vi "Update Conditional Visibility.vi"(10 "Previous UI Data in":refnum<class "Settings UI.lvclass">, 11 "New UI Data in":refnum<class "Settings UI.lvclass">) -> (3 "New UI Data out":refnum<class "Settings UI.lvclass">)   [LabVIEW 2024, in "Output Sequencer.lvlib" / "Settings UI.lvclass"]
uses:
  Settings UI.lvclass
  Types/Tree Index Enum.ctl
  Settings UI.lvclass/Settings UI.ctl
  Globals/Global Tree Data.vi
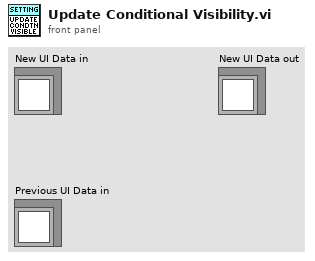
[diagram p1: front panel]
types:
  T1 = typedef "Output Sequencer.lvlib/Settings UI.lvclass/Tree Index Enum.ctl" = enum16{"General Settings", "Num Steps", "Num Analog", "Num Digital", "Show Confirmation", "Interp Priority", "Adv Timing", "Enable Conditions", "Seq Execution", "Reset Test Start", "Only When Test", "Delay After Test", "Start condition", "Re-triggering", "Stop condition", "Stop After Cycles", "Stop Values", "Default Values", "Default Analog", "Default Digital", "Steps", "Step #", "Description", "Precondition", "Duration", "Mode", "Delay Between Vals", "Analog Values", "Digital Values", "Postcondition", "On True", "On False"}
  T2 = typedef "Output Sequencer.lvlib/Settings UI.lvclass/Step Settings.ctl" = cluster{"Description":string, "Precondition":string, "Duration":dbl, "Mode":string, "Delay Between Values":dbl, "Analog Values":string[], "Digital Values":string[], "Postcondition":string, "On True":string, "On False":string}
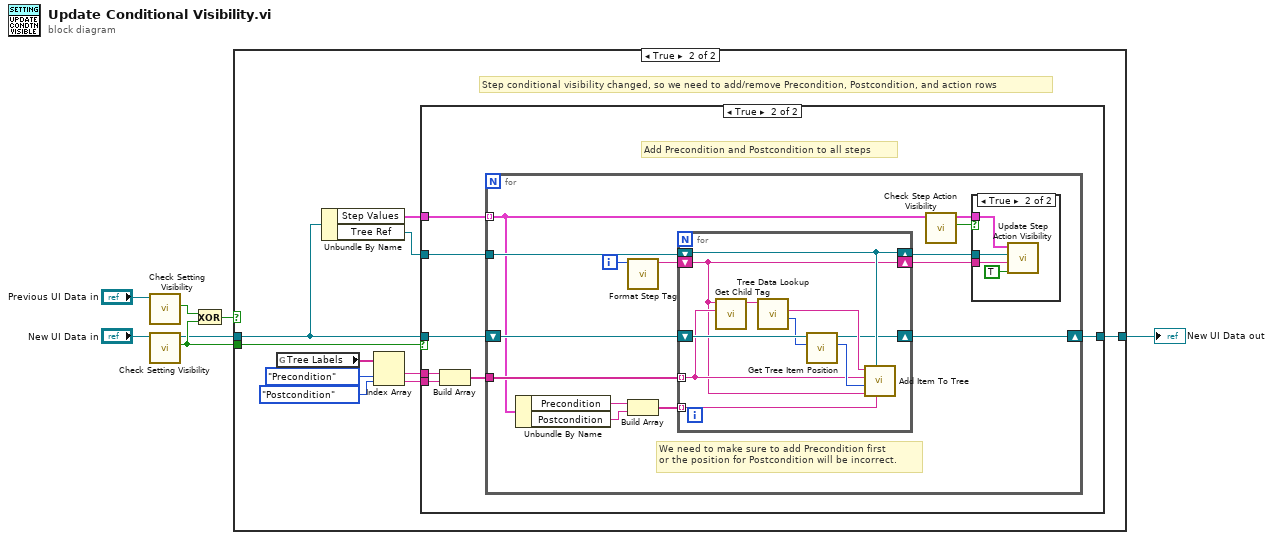
[diagram p0: block diagram]
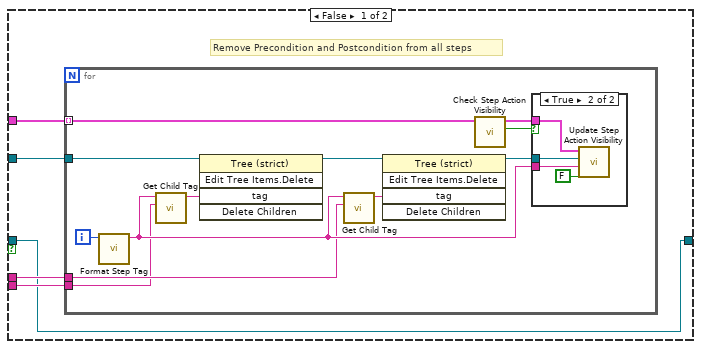
[diagram p3: hidden frame]
diagram:
  n1 = call "Check Setting Visibility.vi"("UI Data in"="Previous UI Data in") -> ("Conditional settings visible"=w3:bool)  [unwired: 7 in, 3 out]
  n2 = call "Check Setting Visibility.vi"("UI Data in"="New UI Data in") -> ("Conditional settings visible"=w4:bool, "UI Data out"=w2:refnum<class "Settings UI.lvclass">)  [unwired: 7 in, 2 out]
  n3 = Exclusive Or(1:w4, 2:w3) -> (0:w7:bool)
  n4 = case shown="True" w7 {
    tunnel: w4 -> [_ w18]
    tunnel: w2 -> [w8 w12]
    tunnel: [w8 w9] -> w1
    frame False {
      # "Change didn't affect if we should or should not display Precondition and Postcondition"
    }
    frame True {
      # "Step conditional visibility changed, so we need to add/remove Precondition, Postcondition, and action rows"
      n5 = global read "Global Tree Data.vi" "Tree Labels"() -> (w17:string[])
      n6 = Unbundle By Name(w12) -> ("Step Values"=w11:T2[], "Tree Ref"=w10:refnum<vi>)
      n7 = Index Array(array=w17, index #1=Tree_Index_Enum."Precondition" ("Tree Index Enum"), index #2=Tree_Index_Enum."Postcondition" ("Tree Index Enum")) -> (element #1=w14:string, element #2=w13:string)
      n8 = case shown="True" w18 {
        tunnel: w10 -> [w23 w46]
        tunnel: w11 -> [w22 w45]
        tunnel: w12 -> [w19 w44]
        tunnel: w14 -> [w21 w43]
        tunnel: w13 -> [w20 w42]
        tunnel: [w19 w40] -> w9
        frame False {
          # "Remove Precondition and Postcondition from all steps"
          n9 = for {
            tunnel: w23 -> [w35]
            tunnel: w22 -> [w31] mode=indexing
            tunnel: w21 -> [w25]
            tunnel: w20 -> [w24]
            i -> [w27]
            n10 = call "Format Step Tag.vi"("Step Number"=w27) -> ("Tag"=w26:string)  [unwired: 10 in]
            n11 = call "Get Child Tag.vi"("Child label"=w24, "Parent tag"=w26) -> ("Child tag"=w29:string)  [unwired: 9 in]
            n12 = invoke class="Tree (strict)" method="Edit Tree Items.Delete"(reference=w35, "tag"=w29) -> (reference out=w34:refnum<vi>)  [unwired: 3 in, 4 out]
            n13 = call "Get Child Tag.vi"("Child label"=w25, "Parent tag"=w26) -> ("Child tag"=w28:string)  [unwired: 9 in]
            n14 = invoke class="Tree (strict)" method="Edit Tree Items.Delete"(reference=w34, "tag"=w28) -> (reference out=w32:refnum<vi>)  [unwired: 3 in, 4 out]
            n15 = call "Check Step Action Visibility.vi"("Step Settings in"=w31) -> ("Actions visible"=w33:bool, "Step Settings out"=w30:T2)  [unwired: 9 in]
            n16 = case shown="True" w33 {
              tunnel: w32 -> [_ w39]
              tunnel: w30 -> [_ w38]
              tunnel: w26 -> [_ w37]
              frame False {
              }
              frame True {
                n17 = call "Update Step Action Visibility.vi"("Actions visible"=FALSE, "Step tag"=w37, "TreeControl in"=w39, "Step Settings"=w38) -> ()  [unwired: 8 in]
              }
            }
          }
        }
        frame True {
          # "Add Precondition and Postcondition to all steps"
          n18 = Build Array(w43, w42) -> (w41:string[])
          n19 = for {
            tunnel: w45 -> [w48] mode=indexing
            tunnel: w41 -> [w55]
            tunnel: w46 -> [w59]
            shift-right: [w47] -> w40
            shift-left: w44 -> [w57]
            i -> [w56]
            # "We need to make sure to add Precondition first\nor the position for Postcondition will be incorrect."
            n20 = Unbundle By Name(w48) -> ("Precondition"=w60:string, "Postcondition"=w54:string)
            n21 = call "Format Step Tag.vi"("Step Number"=w56) -> ("Tag"=w50:string)  [unwired: 10 in]
            n22 = Build Array(w60, w54) -> (w58:string[])
            n23 = for {
              tunnel: w55 -> [w71] mode=indexing
              tunnel: w58 -> [w70] mode=indexing
              shift-right: [w67] -> w51
              shift-left: w59 -> [w67]
              shift-right: [w66] -> w49
              shift-left: w50 -> [w66]
              shift-right: [w65] -> w47
              shift-left: w57 -> [w74]
              n24 = call "Get Child Tag.vi"("Child label"=w71, "Parent tag"=w66) -> ("Child tag"=w69:string)  [unwired: 9 in]
              n25 = call "Tree Data Lookup.vi"("Tag in"=w69) -> ("Tree Index Enum"=w73:T1, "Tag out"=w68:string)  [unwired: 5 in, 4 out]
              n26 = call "Get Tree Item Position.vi"("Step item"=w73, "UI Data in"=w74) -> ("Position"=w72:i32, "UI Data out"=w65:refnum<class "Settings UI.lvclass">)  [unwired: 8 in]
              n27 = call "Add Item To Tree.vi"("Child Text"=w70, "TreeControl in"=w67, "Parent Tag"=w66, "Child Position"=w72, "Left Cell String"=w71, "Child Tag in"=w68) -> ()  [unwired: 5 in, 1 out]
            }
            n28 = call "Check Step Action Visibility.vi"("Step Settings in"=w48) -> ("Actions visible"=w52:bool, "Step Settings out"=w53:T2)  [unwired: 9 in]
            n29 = case shown="True" w52 {
              tunnel: w53 -> [_ w64]
              tunnel: w51 -> [_ w63]
              tunnel: w49 -> [_ w62]
              frame False {
              }
              frame True {
                n30 = call "Update Step Action Visibility.vi"("Actions visible"=TRUE, "Step tag"=w62, "TreeControl in"=w63, "Step Settings"=w64) -> ()  [unwired: 8 in]
              }
            }
          }
        }
      }
    }
  }
  "New UI Data out" <- w1
